vi "_EN1 Installer.vi"() -> ()   [LabVIEW 2019]
panel:
  out "error out":errorcluster
  out "Target Path":path
  out "Source Path":path
  out "folder names":string[](array[string])
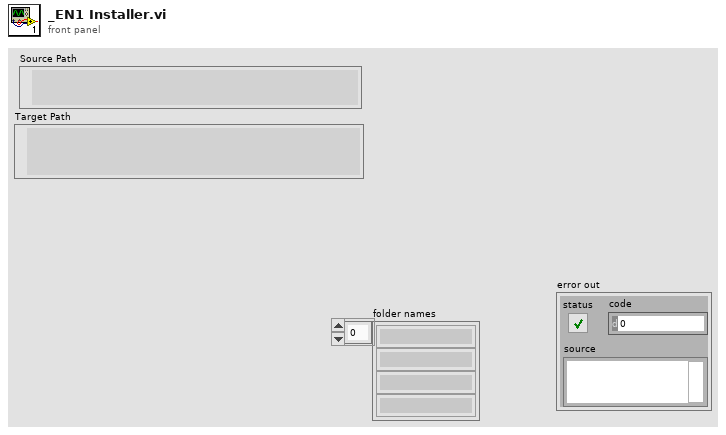
[diagram p1: front panel]
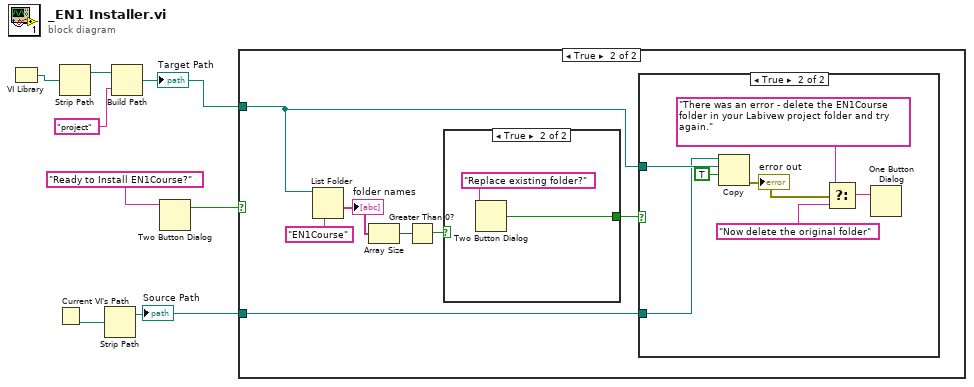
[diagram p0: block diagram]
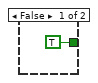
[diagram p4: hidden frame]
diagram:
  n1 = VI Library() -> (path=w5:path)
  n2 = Current VI's Path() -> (path=w2:path)
  n3 = Strip Path(path=w5) -> (stripped path=w6:path)  [unwired: 1 out]
  n4 = Strip Path(path=w2) -> (stripped path=w1:path)  [unwired: 1 out]
  "Source Path" <- w1
  n5 = Build Path(base path=w6, name or relative path="project") -> (appended path=w3:path)
  "Target Path" <- w3
  n6 = Two Button Dialog(message="Ready to Install EN1Course?") -> (T button?=w7:bool)  [unwired: 2 in]
  n7 = case shown="True" w7 {
    tunnel: w3 -> [_ w10]
    tunnel: w1 -> [_ w9]
    frame False {
    }
    frame True {
      n8 = List Folder(path=w10, pattern="EN1Course") -> (folder names=w14:string[])  [unwired: 2 in, 3 out]
      "folder names" <- w14
      n9 = Array Size(array=w14) -> (size(s)=w13:i32)
      n10 = Greater Than 0?(x=w13) -> (x > 0?=w12:bool)
      n11 = case shown="True" w12 {
        tunnel: [TRUE ("T button?") w24] -> w11
        frame False {
        }
        frame True {
          n12 = Two Button Dialog(message="Replace existing folder?") -> (T button?=w24:bool)  [unwired: 2 in]
        }
      }
      n13 = case shown="True" w11 {
        tunnel: w10 -> [_ w22]
        tunnel: w9 -> [_ w21]
        frame False {
        }
        frame True {
          n14 = Copy(9:TRUE ("overwrite (F)"), 10:w22, 11:w21) -> (0:w19:errorcluster)  [unwired: 2 in, 2 out]
          "error out" <- w19
          n15 = Select(t="There was an error - delete the EN1Course folder in your Labivew project folder and try again." ("message"), s=w19, f="Now delete the original folder" ("message")) -> (s? t:f=w16:string)
          n16 = One Button Dialog(message=w16) -> ()  [unwired: 1 in, 1 out]
        }
      }
    }
  }
